vi "Pack.vi"(8 "error in":errorcluster, 10 "destination folder":path, 11 "source folder":path) -> (0 "error out":errorcluster, 3 "package filepath":path)   [LabVIEW 2014, in "NIPM_API.lvlib"]
doc: "Creates or packs a package"
uses:
  NIPM_API.lvlib
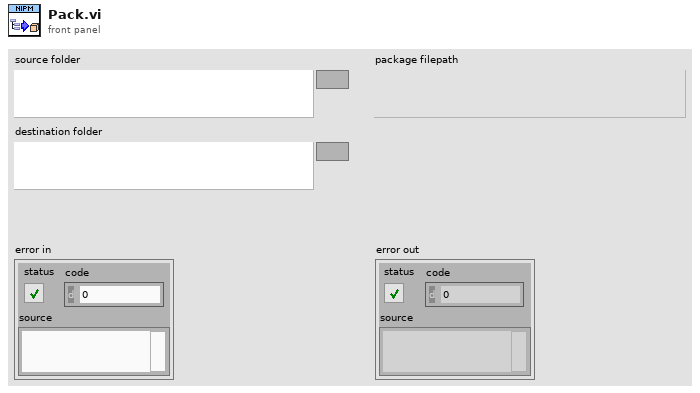
[diagram p1: front panel]
types:
  T1 = typedef "NIPM_API.lvlib/package attributes.ctl" = cluster{"Package Name":string, "Display name":string, "Version":string, "Display version":string, "Synopsis":string, "Description":string, "Maintainer":string, "Maintainer email address":string, "Category":string, "Homepage":string, "Release notes":string, "Depends":string[], "Recommends":string[], "Suggests":string[], "Conflicts":string[], "Provides":string[], "Replaces":string[], "Supplements":string[], "Enhances":string[], "Product":bool, "User visible":bool, "Installed size (KB)":u64, "Package filesize (bytes)":u64, "Architecture":string, "Agent":string, "MD5Checksum":string}
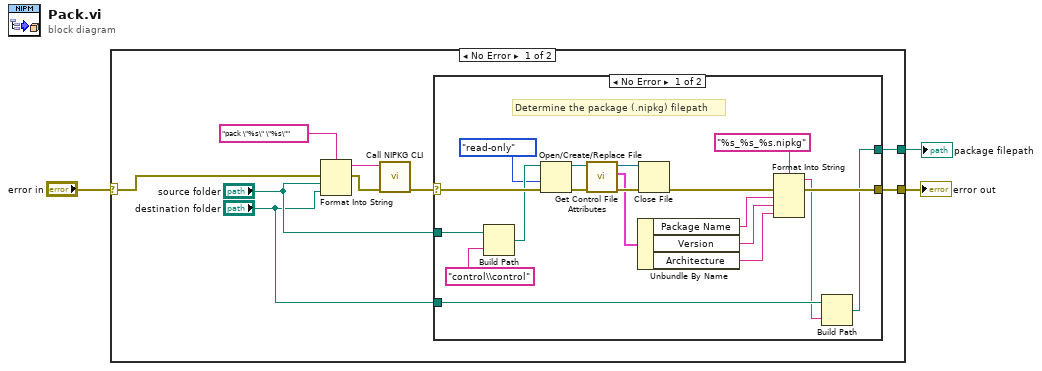
[diagram p0: block diagram]
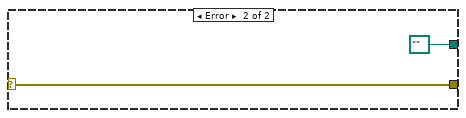
[diagram p2: hidden frame]
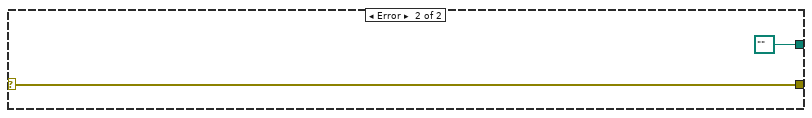
[diagram p3: hidden frame]
diagram:
  n1 = case shown="No Error" "error in" {
    selector: "error in" -> [w11 w35]
    tunnel: [w5 w35] -> w2
    tunnel: [w4 path "" ("appended path")] -> w1
    frame No Error {
      n2 = Format Into String(format string="pack \"%s\" \"%s\"", error in=w11, "source folder", "destination folder") -> (resulting string=w9:string, error out=w10:errorcluster)  [unwired: 1 in]
      n3 = call "Call NIPKG CLI.vi"("error in (no error)"=w10, "command"=w9) -> ("error out"=w8:errorcluster)  [unwired: 8 in, 1 out]
      n4 = case shown="No Error" w8 {
        selector: w8 -> [w29 w33]
        tunnel: "source folder" -> [w31 _]
        tunnel: "destination folder" -> [w21 _]
        tunnel: [w15 w33] -> w5
        tunnel: [w13 path "" ("appended path")] -> w4
        frame No Error {
          # "Determine the package (.nipkg) filepath"
          n5 = Build Path(base path=w31, name or relative path="control\\control") -> (appended path=w28:path)
          n6 = Open/Create/Replace File(file path (use dialog)=w28, error in=w29, access (0:read/write)=enum16{"read/write", "read-only", "write-only"}."read-only") -> (refnum out=w26:refnum<file>, error out=w25:errorcluster)  [unwired: 3 in, 1 out]
          n7 = call "Get Control File Attributes.vi"("error in (no error)"=w25, "control file refnum in"=w26) -> ("error out"=w24:errorcluster, "package attributes"=w22:T1, "control file refnum out"=w23:refnum<file>)  [unwired: 7 in]
          n8 = Unbundle By Name(w22) -> ("Package Name"=w18:string, "Version"=w17:string, "Architecture"=w16:string)
          n9 = Close File(refnum=w23, error in=w24) -> (error out=w19:errorcluster)  [unwired: 1 out]
          n10 = Format Into String(format string="%s_%s_%s.nipkg", error in=w19, w18, w17, w16) -> (resulting string=w14:string, error out=w15:errorcluster)  [unwired: 1 in]
          n11 = Build Path(base path=w21, name or relative path=w14) -> (appended path=w13:path)
        }
        frame Error {
        }
      }
    }
    frame Error {
    }
  }
  "error out" <- w2
  "package filepath" <- w1
